vi "VICI_LRN.vi"() -> ()   [LabVIEW 2023]
panel:
  out "read buffer":string
  out "error out":errorcluster
  in  "Valve COM":refnum<visa-resource-name>="COM8"
  in  "Valve ID":string="1"
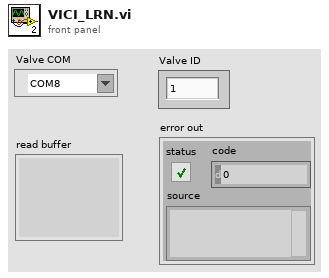
[diagram p1: front panel]
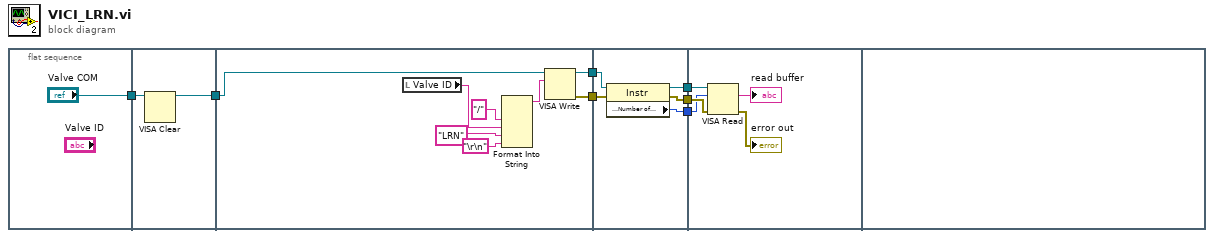
[diagram p0: block diagram]
diagram:
  n1 = flat-sequence {
    tunnel: ["Valve COM"] -> w7
    tunnel: w7 -> [w10]
    tunnel: [w9] -> w6
    tunnel: [w14] -> w5
    tunnel: [w13] -> w4
    tunnel: w6 -> [w12]
    tunnel: w5 -> [w23]
    tunnel: [w21] -> w3
    tunnel: w4 -> [w22]
    tunnel: [w20] -> w2
    tunnel: [w19] -> w1
    tunnel: w3 -> [w28]
    tunnel: w2 -> [w27]
    tunnel: w1 -> [w26]
    frame #0 {
    }
    frame #1 {
      n2 = VISA Clear(VISA resource name=w10) -> (VISA resource name out=w9:refnum<visa-resource-name>)  [unwired: 1 in, 1 out]
    }
    frame #2 {
      n3 = local read "Valve ID"() -> (w18:string)
      n4 = Format Into String("/", w18, "LRN", "\r\n") -> (resulting string=w15:string)  [unwired: 3 in, 1 out]
      n5 = VISA Write(VISA resource name=w12, write buffer=w15) -> (VISA resource name out=w14:refnum<visa-resource-name>, error out=w13:errorcluster)  [unwired: 1 in, 1 out]
    }
    frame #3 {
      n6 = property class="Instr"(reference=w23, error in=w22) -> (reference out=w21:refnum<visa-resource-name>, error out=w20:errorcluster, "Serial Settings:Number of Bytes at Serial Port"=w19:u32)
    }
    frame #4 {
      n7 = VISA Read(VISA resource name=w28, byte count=w26, error in (no error)=w27) -> (read buffer=→"read buffer":string, error out=→"error out":errorcluster)  [unwired: 2 out]
    }
    frame #5 {
    }
  }
